vi "1L02-cumul1D.vi"(4 "som_X":u32, 7 "X":dbl[](array[numeric])=[3.0, 5.0, 14.0, 12.0, 22.0, 20.0, 16.0, 3.0, 5.0]) -> (0 "som_X":u32, 1 "X cum en %":dbl[](array[numeric]), 2 "X en %":dbl[](array[numeric]), 3 "X Cum":dbl[](array[numeric]))   [LabVIEW 2010, in "lv_01.lvlib"]
doc: "A partir d'une série X, on calcule les données suivants :\n- X cum : valeurs de X cumulées\n- X en % : pourcentage des valeurs de X relative à som_X\n- X cum en % : valeurs de X cumulées en % relatives à som_X\nSi som_X est absent ou nul, alors som_X est initialisé avec la somme des valeurs X"
uses:
  lv_01.lvlib
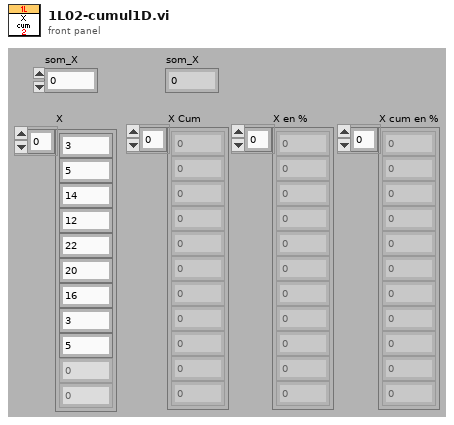
[diagram p1: front panel]
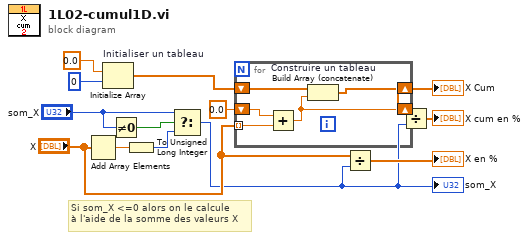
[diagram p0: block diagram]
diagram:
  # "Si som_X <=0 alors on le calcule\nà l'aide de la somme des valeurs X"
  n1 = Add Array Elements(numeric array="X") -> (sum=w11:dbl)
  n2 = Initialize Array "Initialiser un tableau"(0.0 ("élément"), 0 ("taille de la dimension")) -> (w6:dbl[])
  n3 = Not Equal To 0?(x="som_X") -> (x != 0?=w13:bool)
  n4 = To Unsigned Long Integer(number=w11) -> (unsigned 32bit integer=w10:u32)
  n5 = Select(t="som_X", s=w13, f=w10) -> (s? t:f=w1:u32)
  "som_X" <- w1
  n6 = for {
    tunnel: "X" -> [w18] mode=indexing
    shift-right: [w16] -> w3
    shift-left: w6 -> [w15]
    shift-right: [w14] -> _
    shift-left: 0.0 -> [w17]
    n7 = Add(x=w17, y=w18) -> (x+y=w14:dbl)
    n8 = Build Array (concatenate) "Construire un tableau"(w15, w14) -> (w16:dbl[])
  }
  "X Cum" <- w3
  n9 = Divide(x="X", y=w1) -> (x/y=→"X en %":dbl[])
  n10 = Divide(x=w3, y=w1) -> (x/y=→"X cum en %":dbl[])
